vi "mqttTCPIPReadRemainingByteQuantity.vi"(8 "error in (no error)":errorcluster, 9 "readTimeout ms (2000)":i32=2000, 10 "remainingLengthByte1":u8 format="%08b", 11 "connRef in":refnum<k5>) -> (0 "error out":errorcluster, 2 "remainingLength":i32, 3 "connRef out":refnum<k5>)   [LabVIEW 2020, in "mqtt.lvclass"]
uses:
  mqtt.lvclass
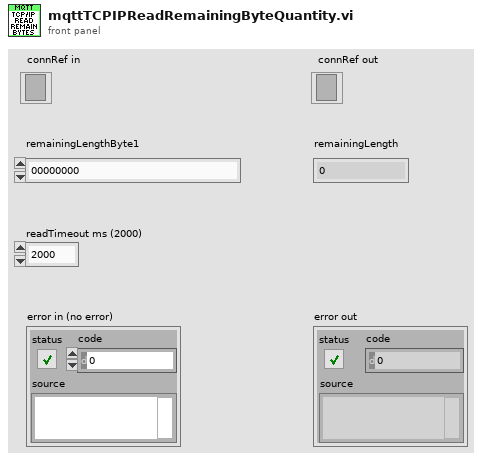
[diagram p1: front panel]
types:
  T1 = enum16{"Standard", "Buffered", "CRLF", "Immediate"}
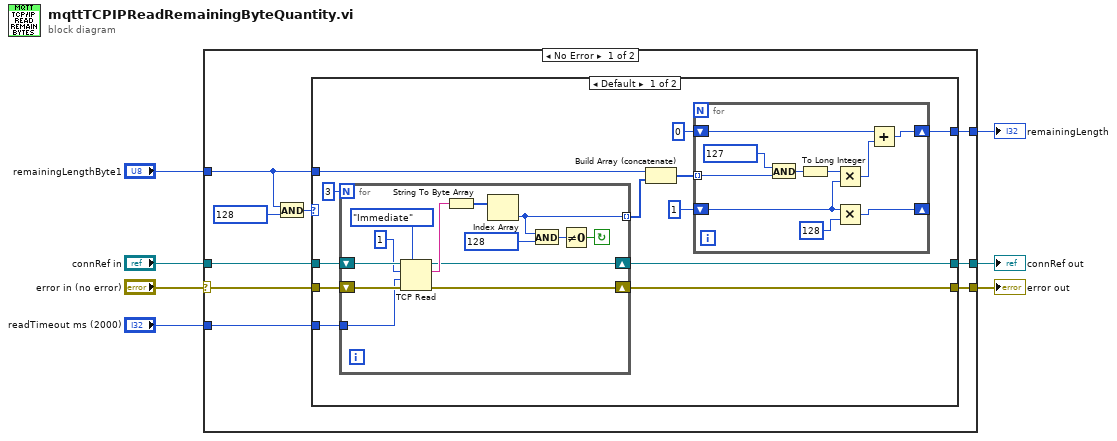
[diagram p0: block diagram]
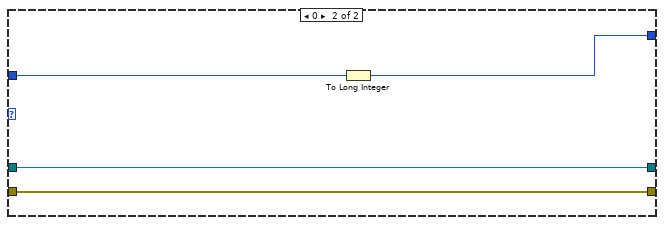
[diagram p2: hidden frame]
diagram:
  n1 = case shown="No Error" "error in (no error)" {
    selector: "error in (no error)" -> [w9 w56]
    tunnel: [w14 _] -> w7
    tunnel: "remainingLengthByte1" -> [w13 _]
    tunnel: "connRef in" -> [w12 w57]
    tunnel: [w11 w57] -> w4
    tunnel: [w10 w56] -> w3
    tunnel: "readTimeout ms (2000)" -> [w8 _]
    frame No Error {
      n2 = And(x=w13, y=u8 128) -> (x .and. y?=w15:u8)
      n3 = case shown="Default" w15 {
        tunnel: [w22 w53] -> w14
        tunnel: w13 -> [w26 w55]
        tunnel: w12 -> [w28 w54]
        tunnel: [w27 w54] -> w11
        tunnel: [w19 w52] -> w10
        tunnel: w9 -> [w18 w52]
        tunnel: w8 -> [w17 _]
        frame Default {
          n4 = for {
            N: 3 -> [_]
            shift-right: [w38] -> w27
            shift-left: w28 -> [w41]
            tunnel: [w35] -> w24 mode=indexing
            shift-right: [w32] -> w19
            shift-left: w18 -> [w31]
            tunnel: w17 -> [w29]
            stop <- w33 continue-if-true
            n5 = TCP Read(connection ID=w41, bytes to read=1, error in (no error)=w31, 7:T1."Immediate" ("mode (standard)"), 9:w29) -> (connection ID out=w38:refnum<k5>, data out=w39:string, error out=w32:errorcluster)
            n6 = String To Byte Array(string=w39) -> (unsigned byte array=w37:u8[])
            n7 = Index Array(array=w37) -> (element=w35:u8)  [unwired: 1 in]
            n8 = And(x=w35, y=u8 128) -> (x .and. y?=w34:u8)
            n9 = Not Equal To 0?(x=w34) -> (x != 0?=w33:bool)
          }
          n10 = Build Array (concatenate)(w26, w24) -> (w21:u8[])
          n11 = for {
            tunnel: w21 -> [w51] mode=indexing
            shift-right: [w47] -> w22
            shift-left: 0 -> [w46]
            shift-right: [w42] -> _
            shift-left: 1 -> [w43]
            n12 = And(x=u8 127 ("y"), y=w51) -> (x .and. y?=w49:u8)
            n13 = To Long Integer(number=w49) -> (32bit integer=w48:i32)
            n14 = Multiply(x=w48, y=w43) -> (x*y=w45:i32)
            n15 = Multiply(x=w43, y=128 ("x")) -> (x*y=w42:i32)
            n16 = Add(x=w46, y=w45) -> (x+y=w47:i32)
          }
        }
        frame 0 {
          n17 = To Long Integer(number=w55) -> (32bit integer=w53:i32)
        }
      }
    }
    frame Error {
    }
  }
  "remainingLength" <- w7
  "connRef out" <- w4
  "error out" <- w3
